vi "MA3 Demonstrator w Help.vi"() -> ()   [LabVIEW 2015]
doc: "MA3 Demonstrator w Help\nThe 'Enc Sim' control simulates the encoder position (six full revolutions) in order to test the MA3 Revolutions subVI."
uses:
  <vilib>/addons/control/pid/pid.llb/PID Output Rate Limiter (DBL).vi
  <vilib>/addons/control/pid/NI_PID_pid.lvlib
panel:
  out "max safe sampling rate (ms)":dbl
  out "Rev/sec":dbl
  out "max":dbl
  in  "loop period (ms)":u32=25
  in  "V/sec":dbl=80.0 format="%.2f"
  out "peak adjacent (V)":dbl
  out "noise peak (V)":dbl
  out "Revs 2":dbl(knob) scale=-10.0..10.0
  in  "noise level (V)":dbl(knob)=0.24973505784301464 scale=0.0..1.0
  out "Revs":dbl
  in  "CW is Up":bool=TRUE
  in  "Enc Sim":dbl(slide) scale=0.0..30.0
  # "Cross-over detector can not\nbe spoofed if this value is kept\nbelow the discriminant (2.5)."
  # "CCW"
  # "CW"
  # "The 'Enc Sim' control simulates the encoder position (six \nfull revolutions) in order to test the MA3 Revolutions \nsubVI.  Since the subVI depends on sucessive readings, \nthis simulator rate limits the control input to accurately \nreflect the behavior of an actual encoder's maximum \nrate of change.\n\n'Revs' and 'Revs 2' indicate the subVI output.\nNote that the 'noise level' control can be used to \nintroduce noise on the simulated signal, to evaluate\nsubVI tolerance to noise.  Although the noise will pass\nthrough to the output, it will not spoof the subVIs\ncrossover detector until it peaks at 1/4th of the sensor's\nrange - or 1.25 volts, when sensor is not moving.  It is \nnot normal for the actual noise level to ever be this high,\n(if so check wiring), so the subVI should reliably report \nencoder position in the presence of noise.\n\nSet 'CW is Up' to True if increasing sensor voltage is to\nrepresent increasing revolutions.  Set to False if voltage\nand revolutions are negatively correlated.  Notice the zero\nreference postion is the Rev=1 position when 'CW is Up'\nis False."
  # "The sum of peak-to-peak noise (2*n) and the product of\nthe max sensor rate of change and the loop period \nmust be less than the discriminant (2.5V) to prevent the \ncross-over detector from false detects.  The max sensor\nrate of change is the 'V/sec' control.  Try setting 'noise \nlevel', 'V/sec', and 'loop period' to values simulating\nintended operations.   Instead of dragging the 'Enc Sim'\ncontrol, just click a new position to cause the simulated\nsensor to change at the maximum selected rate. Notice \nthat as long as the 'loop  period' is kept less than 'max \nsafe sampling rate', the subVI will work reliably, but will \nfalsely detect range cross-overs when 'loop period' is \ntoo long.  When the loop period is too long for a given\nnoise level and sensor rate of change, the subVI output\nmay go backwards or become erratic as it begins to\ncount range cross-overs that did not actually occur."
  # "For reliable operation, the loop period must be fast enough ...\n\n                             Loop Period < (2.5 - 2*n) / (5 * Sensor RPS)\nwhere:\n                             n = peak noise level, in volts\n                             Sensor RPS = maximum rate the sensor might change, in revolutions per second\n                             Loop Period = minimum required sampling rate of sensor, in seconds"
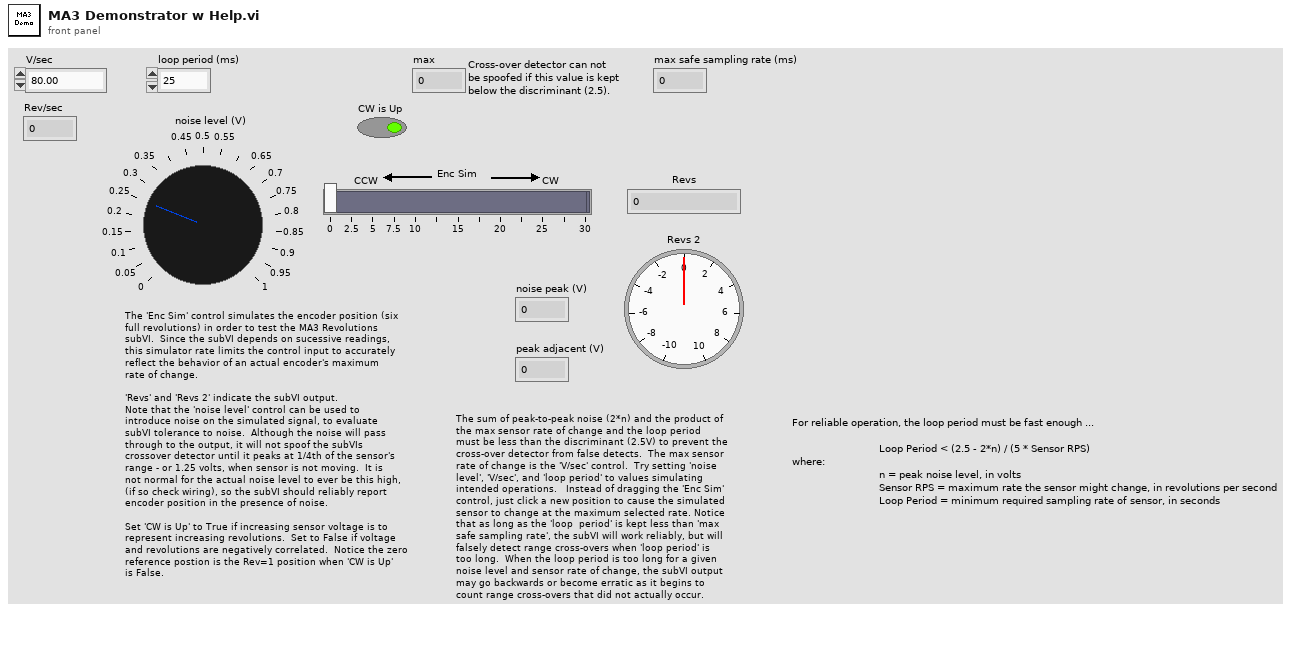
[diagram p1: front panel]
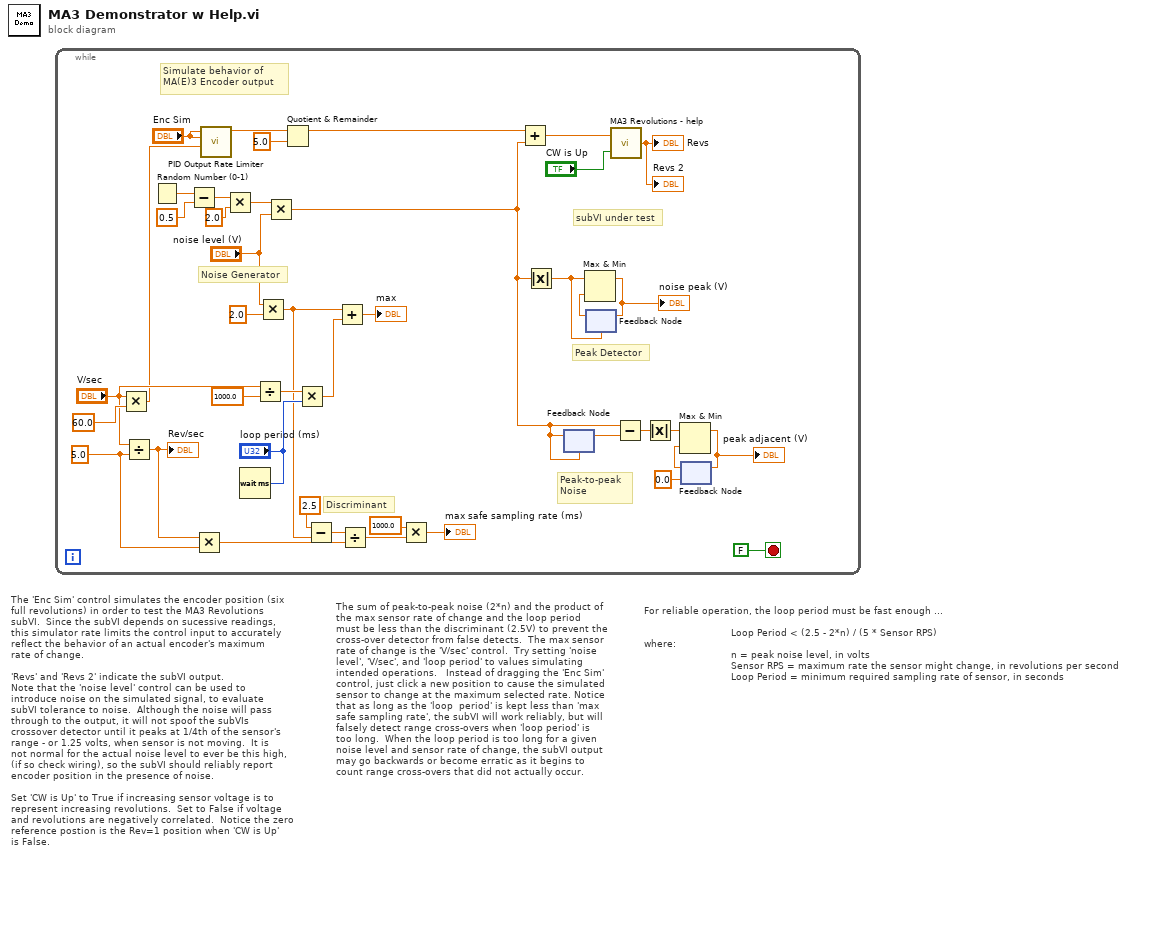
[diagram p0: block diagram]
diagram:
  # "For reliable operation, the loop period must be fast enough ...\n\n                             Loop Period < (2.5 - 2*n) / (5 * Sensor RPS)\nwhere:\n                             n = peak noise level, in volts\n                             Sensor RPS = maximum rate the sensor might change, in revolutions per second\n                             Loop Period = minimum required sampling rate of sensor, in seconds"
  # "The sum of peak-to-peak noise (2*n) and the product of\nthe max sensor rate of change and the loop period \nmust be less than the discriminant (2.5V) to prevent the \ncross-over detector from false detects.  The max sensor\nrate of change is the 'V/sec' control.  Try setting 'noise \nlevel', 'V/sec', and 'loop period' to values simulating\nintended operations.   Instead of dragging the 'Enc Sim'\ncontrol, just click a new position to cause the simulated\nsensor to change at the maximum selected rate. Notice \nthat as long as the 'loop  period' is kept less than 'max \nsafe sampling rate', the subVI will work reliably, but will \nfalsely detect range cross-overs when 'loop period' is \ntoo long.  When the loop period is too long for a given\nnoise level and sensor rate of change, the subVI output\nmay go backwards or become erratic as it begins to\ncount range cross-overs that did not actually occur."
  # "The 'Enc Sim' control simulates the encoder position (six \nfull revolutions) in order to test the MA3 Revolutions \nsubVI.  Since the subVI depends on sucessive readings, \nthis simulator rate limits the control input to accurately \nreflect the behavior of an actual encoder's maximum \nrate of change.\n\n'Revs' and 'Revs 2' indicate the subVI output.\nNote that the 'noise level' control can be used to \nintroduce noise on the simulated signal, to evaluate\nsubVI tolerance to noise.  Although the noise will pass\nthrough to the output, it will not spoof the subVIs\ncrossover detector until it peaks at 1/4th of the sensor's\nrange - or 1.25 volts, when sensor is not moving.  It is \nnot normal for the actual noise level to ever be this high,\n(if so check wiring), so the subVI should reliably report \nencoder position in the presence of noise.\n\nSet 'CW is Up' to True if increasing sensor voltage is to\nrepresent increasing revolutions.  Set to False if voltage\nand revolutions are negatively correlated.  Notice the zero\nreference postion is the Rev=1 position when 'CW is Up'\nis False."
  n1 = while {
    stop <- FALSE stop-if-true
    w8 = 5.0 ("y")
    # "Discriminant"
    # "subVI under test"
    # "Peak-to-peak\nNoise"
    # "Noise Generator"
    # "Peak Detector"
    # "Simulate behavior of\nMA(E)3 Encoder output"
    n2 = Multiply(x="V/sec", y=60.0) -> (x*y=w6:dbl)
    n3 = Divide(x="V/sec", y=w8) -> (x/y=w9:dbl)
    "Rev/sec" <- w9
    n4 = Random Number (0-1)() -> (number: 0 to 1=w38:dbl)
    n5 = Subtract(x=w38, y=0.5) -> (x-y=w20:dbl)
    n6 = Multiply(x=w9, y=w8) -> (x*y=w7:dbl)
    n7 = call-poly <vilib>:"PID Output Rate Limiter.vi"("output rate (EGU/min)"=w6, "initial output"="Enc Sim", "input (controller output)"="Enc Sim") -> ("output"=w25:dbl)  [unwired: 5 in, 1 out]
    n8 = Multiply(x=w20, y=2.0) -> (x*y=w19:dbl)
    n9 = Wait (ms)(milliseconds to wait="loop period (ms)") -> ()  [unwired: 1 out]
    n10 = Divide(x="V/sec", y=1000.0) -> (x/y=w23:dbl)
    n11 = Multiply(x="noise level (V)", y=2.0) -> (x*y=w12:dbl)
    n12 = Multiply(x=w19, y="noise level (V)") -> (x*y=w5:dbl)
    n13 = Quotient & Remainder(x=w25, y=5.0) -> (x-y*floor(x/y)=w27:dbl)  [unwired: 1 out]
    n14 = Multiply(x=w23, y="loop period (ms)") -> (x*y=w13:dbl)
    n15 = Subtract(x=2.5, y=w12) -> (x-y=w11:dbl)
    n16 = Add(x=w12, y=w13) -> (x+y=→"max":dbl)
    n17 = Divide(x=w11, y=w7) -> (x/y=w4:dbl)
    n18 = Multiply(x=1000.0, y=w4) -> (x*y=→"max safe sampling rate (ms)":dbl)
    n19 = Add(x=w27, y=w5) -> (x+y=w1:dbl)
    n20 = Absolute Value(x=w5) -> (abs(x)=w33:dbl)
    n21 = feedback-in #1(w5) -> ()
    n22 = feedback #1(w5) -> (w34:dbl)
    n23 = feedback #2(w33) -> (w35:dbl)
    n24 = Max & Min(x=w33, y=w35) -> (max(x,y)=w36:dbl)  [unwired: 1 out]
    "noise peak (V)" <- w36
    n25 = feedback-in #2(w36) -> ()
    n26 = call <userlib>:"MA3 Revolutions - help.vi"("CW is Up"="CW is Up", "V in"=w1) -> ("Revs"=→"Revs" →"Revs 2":dbl)
    n27 = Subtract(x=w5, y=w34) -> (x-y=w32:dbl)
    n28 = Absolute Value(x=w32) -> (abs(x)=w30:dbl)
    n29 = feedback #3(0.0) -> (w29:dbl)
    n30 = Max & Min(x=w30, y=w29) -> (max(x,y)=w31:dbl)  [unwired: 1 out]
    "peak adjacent (V)" <- w31
    n31 = feedback-in #3(w31) -> ()
  }
